vi "BottomBar.vi"() -> ()   [LabVIEW 2013]
uses:
  nav-button.ctl
  <vilib>/Utility/miscctls.llb/LVPointTypeDef.ctl
  Globals.vi
panel:
  out "array":bool[](array[boolean])
  in  "Buttons":T2
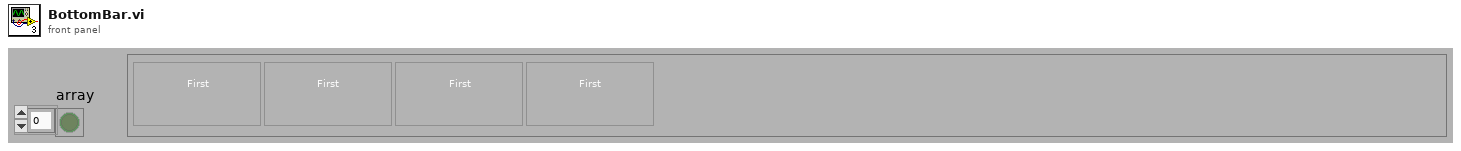
[diagram p1: front panel]
types:
  T1 = typedef "nav-button.ctl" = bool
  T2 = cluster{"OK Button":T1, "OK Button 2":T1, "OK Button 3":T1, "OK Button 5":T1, "OK Button 6":bool, "OK Button 7":bool, "OK Button 8":bool, "OK Button 9":bool, "OK Button 10":bool, "OK Button 4":T1, "OK Button 11":T1, "OK Button 12":T1, "OK Button 13":T1, "OK Button 14":T1, "OK Button 15":T1, "OK Button 16":T1, "OK Button 17":T1, "OK Button 18":T1}
  T3 = typedef "LVPointTypeDef.ctl" = cluster{"Horizontal":i16, "Vertical":i16}
  T4 = typedef "LVAllMonitorsDisplayTypeDef.ctl" = cluster{"Bounds":cluster{"Left":i16, "Top":i16, "Right":i16, "Bottom":i16}, "Depth":i16}[]
  T5 = typedef "LVRectTypeDef.ctl" = cluster{"Left":i16, "Top":i16, "Right":i16, "Bottom":i16}
  T6 = cluster{"Bounds":cluster{"Left":i16, "Top":i16, "Right":i16, "Bottom":i16}, "Depth":i16}
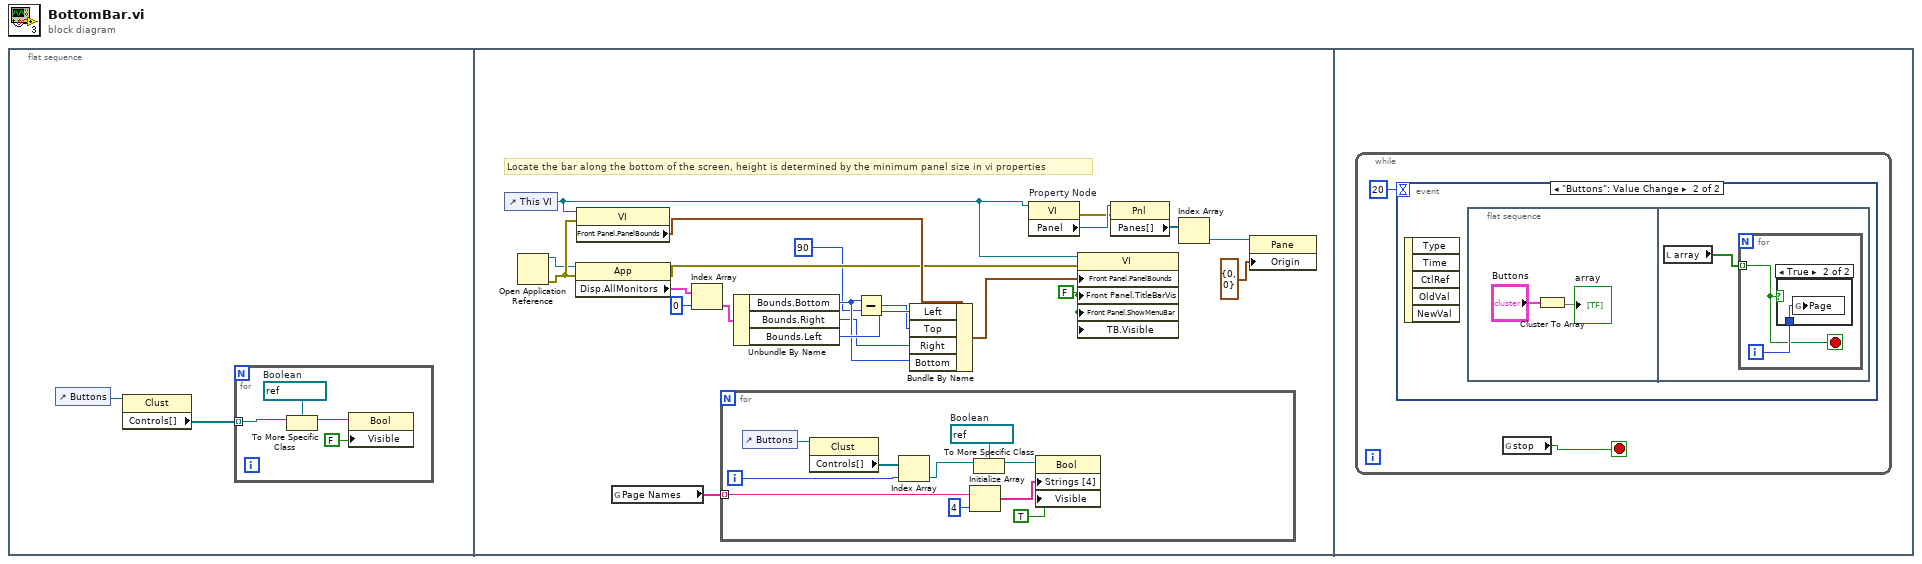
[diagram p0: block diagram]
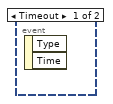
[diagram p2: hidden frame]
diagram:
  n1 = flat-sequence {
    frame #0 {
      n2 = control-ref of="Buttons"() -> (w2:refnum<vi>)
      n3 = property class="Clust"(reference=w2) -> ("Controls[]"=w1:refnum<vi>[])  [unwired: 1 in, 2 out]
      n4 = for {
        tunnel: w1 -> [w3] mode=indexing
        w4 = refnum<vi> refnum  # Boolean
        n5 = To More Specific Class(target class=w4, reference=w3) -> (specific class reference=w5:refnum<vi>)  [unwired: 1 in, 1 out]
        n6 = property class="Bool"(reference=w5, "Visible"=FALSE) -> ()  [unwired: 1 in, 2 out]
      }
    }
    frame #1 {
      w8 = FALSE ("Front Panel Window:Title Bar Visible")
      # "Locate the bar along the bottom of the screen, height is determined by the minimum panel size in vi properties"
      n7 = control-ref of="This VI"() -> (w10:refnum<vi>)
      n8 = Open Application Reference() -> (0:w27:errorcluster, 3:w26:refnum<vi>)  [unwired: 4 in]
      n9 = property class="App"(reference=w26, error in=w27) -> (error out=w19:errorcluster, "Disp.AllMonitors"=w17:T4)  [unwired: 1 out]
      n10 = property class="VI"(reference=w10, error in=w27) -> ("Front Panel.PanelBounds"=w21:T5)  [unwired: 2 out]
      n11 = global read "Globals.vi" "Page Names"() -> (w7:string[])
      n12 = Index Array(array=w17, index=0) -> (element=w16:T6)
      n13 = for {
        tunnel: w7 -> [w36] mode=indexing
        i -> [w29]
        w35 = refnum<vi> refnum  # Boolean
        n14 = control-ref of="Buttons"() -> (w37:refnum<vi>)
        n15 = property class="Clust"(reference=w37) -> ("Controls[]"=w31:refnum<vi>[])  [unwired: 1 in, 2 out]
        n16 = Index Array(array=w31, index=w29) -> (element=w30:refnum<vi>)
        n17 = Initialize Array(w36, 4 ("dimension size")) -> (w32:string[])
        n18 = To More Specific Class(target class=w35, reference=w30) -> (specific class reference=w34:refnum<vi>)  [unwired: 1 in, 1 out]
        n19 = property class="Bool"(reference=w34, "Strings [4]"=w32, "Visible"=TRUE) -> ()  [unwired: 1 in, 2 out]
      }
      n20 = Unbundle By Name(w16) -> ("Bounds.Bottom"=w24:i16, "Bounds.Right"=w23:i16, "Bounds.Left"=w25:i16)
      n21 = Subtract(x=w24, y=i16 90) -> (x-y=w22:i16)
      n22 = Bundle By Name(cluster=w21, "Left"=w25, "Top"=w22, "Right"=w23, "Bottom"=w24) -> (w20:T5)
      n23 = property on="Property Node" class="VI"(reference=w10) -> (error out=w14:errorcluster, "Panel"=w15:refnum<vi>)  [unwired: 1 in, 1 out]
      n24 = property class="VI"(reference=w10, error in=w19, "Front Panel.PanelBounds"=w20, "Front Panel.TitleBarVis"=w8, "Front Panel.ShowMenuBar"=w8, "TB.Visible"=w8) -> ()  [unwired: 2 out]
      n25 = property class="Pnl"(reference=w15, error in=w14) -> ("Panes[]"=w13:refnum<vi>[])  [unwired: 2 out]
      n26 = Index Array "Index Array"(array=w13) -> (element=w12:refnum<vi>)  [unwired: 1 in]
      n27 = property class="Pane"(reference=w12, "Origin"=T3 {"Horizontal"=0, "Vertical"=0}) -> ()  [unwired: 1 in, 2 out]
    }
    frame #2 {
      n28 = while {
        stop <- w38 stop-if-true
        n29 = event shown="[1] \"Buttons\": Value Change" {
          selector: _ -> [_ _]
          dyn-events: _ -> [_ _]
          timeout: 20 -> [_ _]
          event Timeout {
            n30 = event-data() -> ()  [unwired: 1 in, 2 out]
          }
          event "Buttons": Value Change {
            n31 = event-data() -> ()  [unwired: 1 in, 5 out]
            n32 = flat-sequence {
              frame #0 {
                n33 = Cluster To Array(cluster="Buttons") -> (array=→"array":T1[])
              }
              frame #1 {
                n34 = local read "array"() -> (w42:bool[])
                n35 = for {
                  tunnel: w42 -> [w43] mode=indexing
                  i -> [w44]
                  stop <- w43 stop-if-true
                  n36 = case shown="True" w43 {
                    tunnel: w44 -> [_ w45]
                    frame False {
                    }
                    frame True {
                      n37 = global write "Globals.vi" "Page"(w45) -> ()
                    }
                  }
                }
              }
            }
          }
        }
        n38 = global read "Globals.vi" "stop"() -> (w38:bool)
      }
    }
  }
